vi "3.0 Discard FPGA ref and Shutdown.vi"(0 "queue out":refnum<queue>) -> ()   [LabVIEW 2010]
uses:
  2-Low Neurons/2-FPGA VI Typedef.ctl
  <vilib>/rvi/interface/nirviReadWriteControl/nirviReadWriteControl.xnode
  FPGA Bitfiles/1Hindbrain.lvbitx
  1-Hindbrain.vi
  <vilib>/rvi/interface/common/niFpgaNodeNameForErrorReporting.ctl
  <vilib>/rvi/errors/niLvFpgaWhatHappensToTopLevelVI.ctl
  <vilib>/rvi/interface/nirviCloseFPGA/nirviCloseFPGA.xnode
  <vilib>/Utility/error.llb/Error Cluster From Error Code.vi
  <vilib>/rvi/errors/niLvFpgaAdjustHostInterfaceError.vi
  <vilib>/FPGAPlugInAG/cRIO-9104/niLvFpga_Close_cRIO-9104.vi
  NiFpgaLv.dll
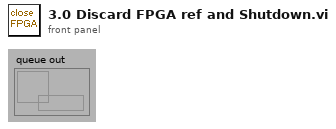
[diagram p1: front panel]
types:
  T1 = typedef "2-FPGA VI Typedef.ctl" = refnum<k20>
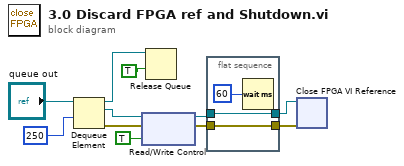
[diagram p0: block diagram]
diagram:
  n1 = Dequeue Element(queue="queue out", timeout in ms (-1)=250) -> (queue out=w7:refnum<queue>, element=w8:T1, error out=w5:errorcluster)  [unwired: 1 in, 1 out]
  n2 = xnode "Read/Write Control"("FPGA VI Reference In"=w8, "error in"=w5, "stop"=TRUE) -> ("FPGA VI Reference Out"=w10:T1, "error out"=w11:errorcluster)
  n3 = Release Queue(queue=w7, force destroy? (F)=TRUE) -> ()  [unwired: 1 in, 3 out]
  n4 = flat-sequence {
    tunnel: w10 -> [w13]
    tunnel: w11 -> [w12]
    tunnel: [w13] -> w3
    tunnel: [w12] -> w4
    frame #0 {
      n5 = Wait (ms)(milliseconds to wait=u32 60) -> ()  [unwired: 1 out]
    }
  }
  n6 = xnode "Close FPGA VI Reference"("FPGA VI Reference In"=w3, "error in"=w4) -> ()  [unwired: 1 out]
